vi "INIConfig(Memory).vi"(8 "error in (no error)":errorcluster, 11 "CSM-Static-Variable-Manager in":refnum<class "CSM-Static-Variable-Manager.lvclass">) -> (0 "error out":errorcluster, 1 "Memory":refnum<class "LabVIEW-Config.lvclass">, 3 "CSM-Static-Variable-Manager out":refnum<class "CSM-Static-Variable-Manager.lvclass">)   [LabVIEW 2017, in "INI-Static-Variable-Support.lvlib" / "CSM-Static-Variable-Manager.lvclass"]
uses:
  CSM-Static-Variable-Manager.lvclass
  LabVIEW-Config/LabVIEW-Config.lvclass
  CSM-Static-Variable-Manager.lvclass/CSM-Static-Variable-Manager.ctl
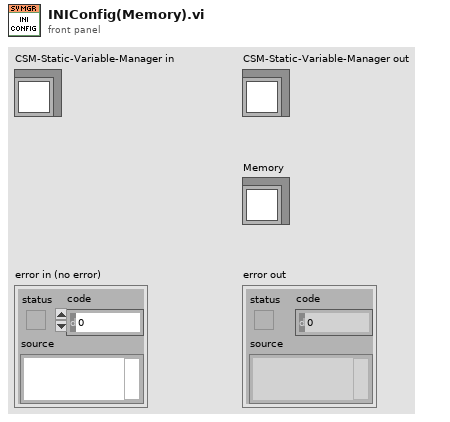
[diagram p1: front panel]
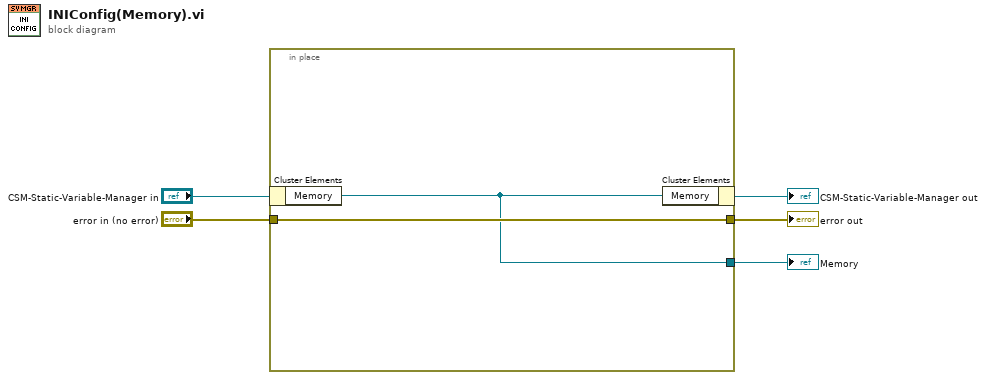
[diagram p0: block diagram]
diagram:
  n1 = in-place {
    in-place-border: "error in (no error)" -> [w7]
    in-place-border: [w7] -> w2
    in-place-border: [w6] -> w1
    n2 = in-place-cluster #1("CSM-Static-Variable-Manager in") -> ("Memory"=w6:refnum<class "LabVIEW-Config.lvclass">)
    n3 = in-place-cluster #1("Memory"=w6) -> (→"CSM-Static-Variable-Manager out":refnum<class "CSM-Static-Variable-Manager.lvclass">)
  }
  "error out" <- w2
  "Memory" <- w1
